vi "rollingAverage_III.vi"(6 "Magnitude Averaging (no. Avgs.)":i32, 9 "785nm":T1, 10 "532nm":T2, 11 "422nm":T3) -> (1 "785nm Data":T5, 2 "532nm Data":T6, 3 "422nm Data":T4)   [LabVIEW 2011]
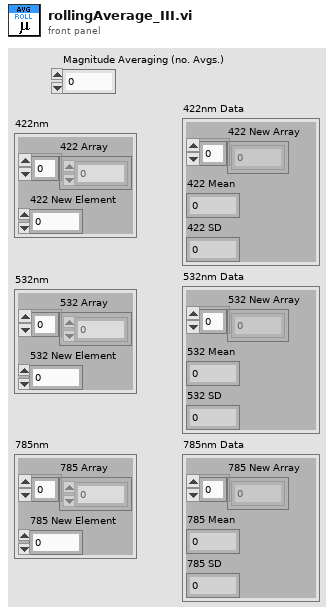
[diagram p1: front panel]
types:
  T1 = cluster{"785 Array":dbl[], "785 New Element":dbl}
  T2 = cluster{"532 Array":dbl[], "532 New Element":dbl}
  T3 = cluster{"422 Array":dbl[], "422 New Element":dbl}
  T4 = cluster{"422 New Array":dbl[], "422 Mean":dbl, "422 SD":dbl}
  T5 = cluster{"785 New Array":dbl[], "785 Mean":dbl, "785 SD":dbl}
  T6 = cluster{"532 New Array":dbl[], "532 Mean":dbl, "532 SD":dbl}
  T7 = cluster{"New Array":dbl[], "mean":dbl, "standard deviation":dbl}
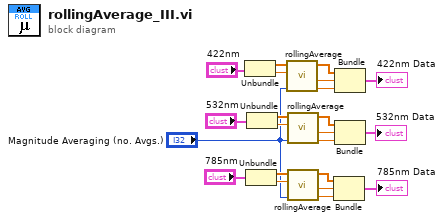
[diagram p0: block diagram]
diagram:
  n1 = Unbundle("422nm") -> ("422 Array"=w17:dbl[], "422 New Element"=w18:dbl)
  n2 = Unbundle("785nm") -> ("785 Array"=w21:dbl[], "785 New Element"=w22:dbl)
  n3 = Unbundle("532nm") -> ("532 Array"=w19:dbl[], "532 New Element"=w20:dbl)
  n4 = call "rollingAverage.vi"("No Avg"="Magnitude Averaging (no. Avgs.)", "New Element"=w18, "Rolling Array"=w17) -> ("standard deviation"=w6:dbl, "mean"=w5:dbl, "New Array"=w16:dbl[])  [unwired: 6 in]
  n5 = call "rollingAverage.vi"("No Avg"="Magnitude Averaging (no. Avgs.)", "New Element"=w20, "Rolling Array"=w19) -> ("standard deviation"=w9:dbl, "mean"=w8:dbl, "New Array"=w7:dbl[])  [unwired: 6 in]
  n6 = call "rollingAverage.vi"("No Avg"="Magnitude Averaging (no. Avgs.)", "New Element"=w22, "Rolling Array"=w21) -> ("standard deviation"=w12:dbl, "mean"=w11:dbl, "New Array"=w10:dbl[])  [unwired: 6 in]
  n7 = Bundle("New Array"=w10, "mean"=w11, "standard deviation"=w12) -> (→"785nm Data":T7)  [unwired: 1 in]
  n8 = Bundle("New Array"=w16, "mean"=w5, "standard deviation"=w6) -> (→"422nm Data":T7)  [unwired: 1 in]
  n9 = Bundle("New Array"=w7, "mean"=w8, "standard deviation"=w9) -> (→"532nm Data":T7)  [unwired: 1 in]
